vi "Station Class Server.vi"() -> ()   [LabVIEW 2018, in "Station.lvclass"]
uses:
  Station.lvclass
  Controls/Server Control.ctl
panel:
  in  "Stop Server":bool
  in  "Delete Ref":bool
  in  "Open References":i32(listbox)
  in  "Lock Server":bool
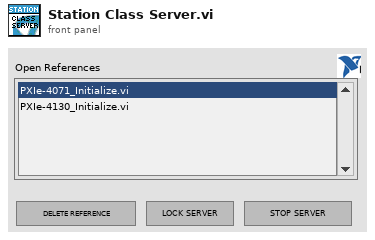
[diagram p1: front panel]
types:
  T1 = typedef "Server Control.ctl" = enum16{"Open New Reference", "Remove Reference", "Kill Server", "Set Station Ref", "Get Station Ref"}
  T2 = cluster{"Action (0: Create)":T1, "Creator Path (=\"\")":path, "Station in":refnum<class "Station.lvclass">}
  T3 = typedef "LVRectTypeDef.ctl" = cluster{"Left":i16, "Top":i16, "Right":i16, "Bottom":i16}
  T4 = cluster{"Action (0: Create)":T1, path, "Station in":refnum<class "Station.lvclass">}
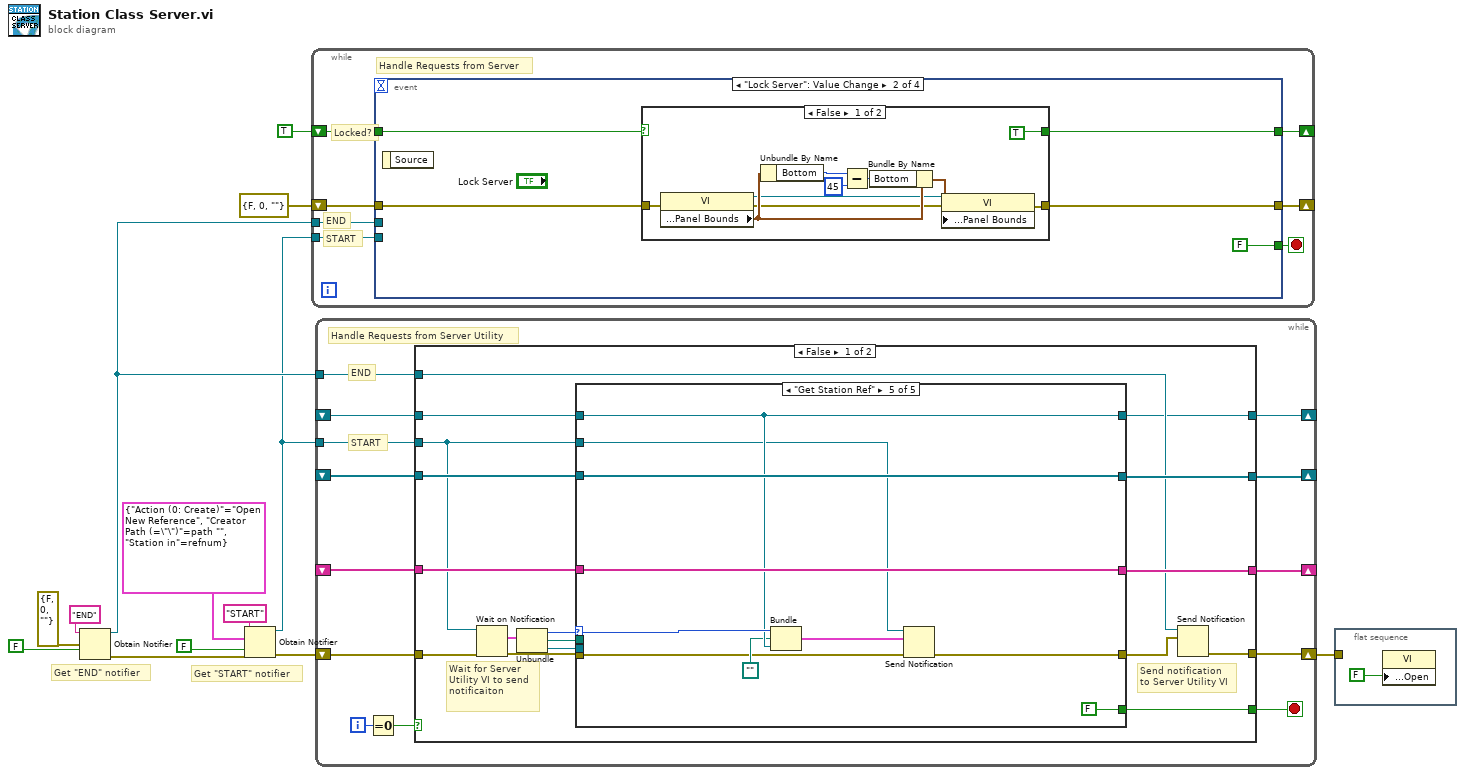
[diagram p0: block diagram]
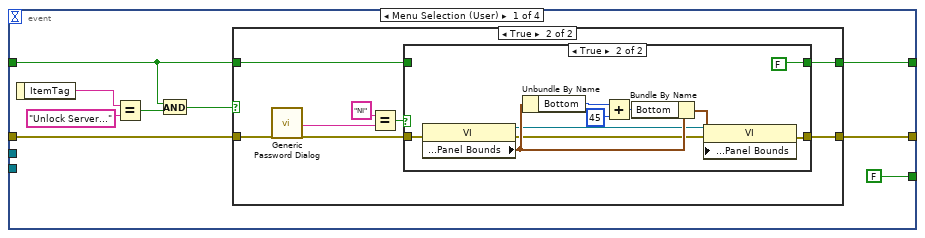
[diagram p2: hidden frame]
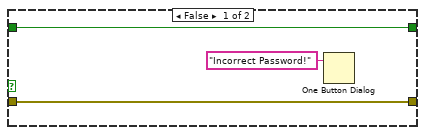
[diagram p4: hidden frame]
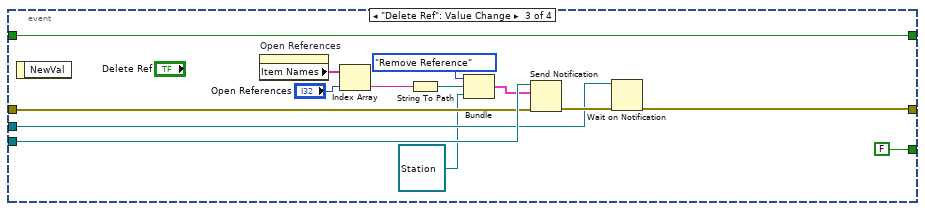
[diagram p6: hidden frame]
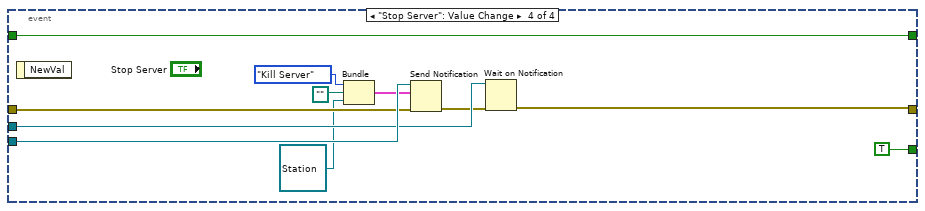
[diagram p7: hidden frame]
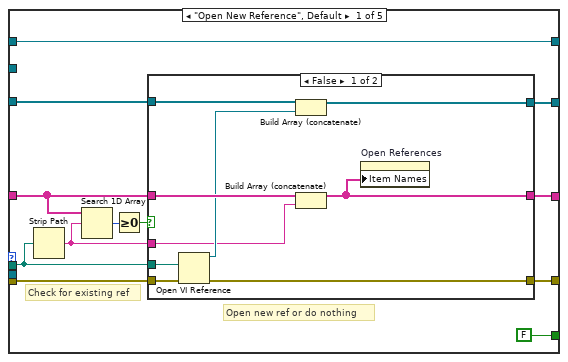
[diagram p8: hidden frame]
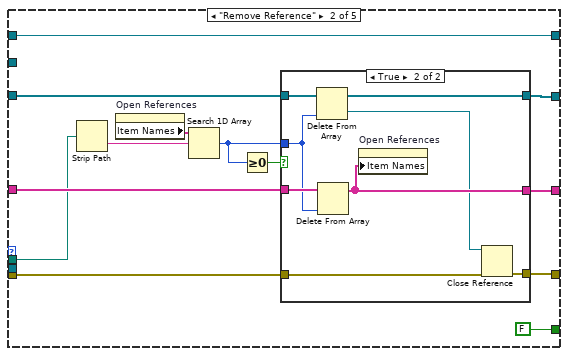
[diagram p10: hidden frame]
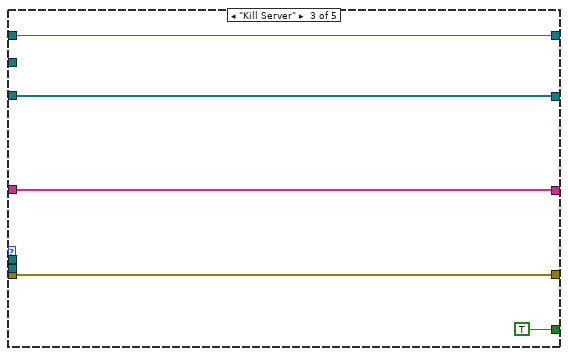
[diagram p12: hidden frame]
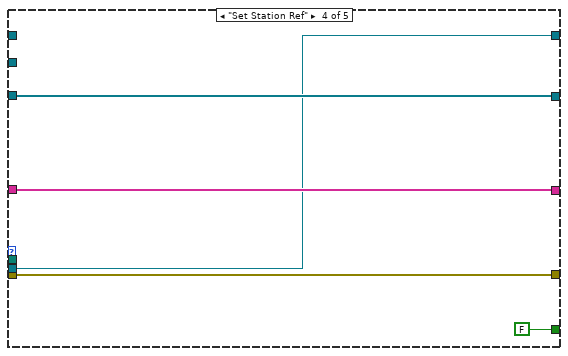
[diagram p13: hidden frame]
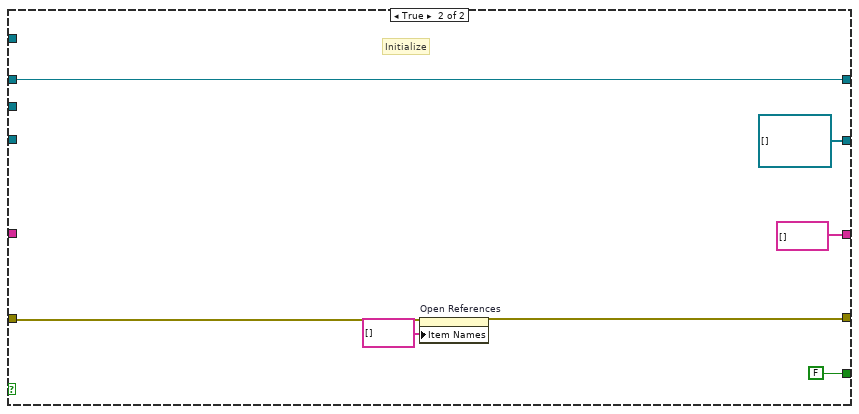
[diagram p14: hidden frame]
diagram:
  # "Get \"START\" notifier"
  # "Get \"END\" notifier"
  n1 = Obtain Notifier(name (unnamed)="END", notification data type=errorcluster {"status"=FALSE, "code"=0, "source"=""} ("error out"), create if not found? (T)=FALSE) -> (notifier out=w6:refnum<notifier>, error out=w7:errorcluster)  [unwired: 1 in, 1 out]
  n2 = Obtain Notifier(name (unnamed)="START", notification data type=T2 {"Action (0: Create)"=enum."Open New Reference", "Creator Path (=\"\")"=path "", "Station in"=refnum} ("output cluster"), create if not found? (T)=FALSE, error in (no error)=w7) -> (notifier out=w1:refnum<notifier>, error out=w5:errorcluster)  [unwired: 1 out]
  n3 = while {
    shift-right: [w18] -> _
    shift-left: errorcluster {"status"=FALSE, "code"=0, "source"=""} ("error out") -> [w19]
    tunnel: w6 -> [w17]
    tunnel: w1 -> [w16]
    shift-right: [w14] -> _
    shift-left: TRUE -> [w15]
    stop <- w20 stop-if-true
    # "Locked?"
    # "Handle Requests from Server"
    # "START"
    # "END"
    n4 = event shown="[1] \"Lock Server\": Value Change" {
      selector: _ -> [_ _ _ _]
      dyn-events: _ -> [_ _ _ _]
      timeout: _ -> [_ _ _ _]
      tunnel: [FALSE FALSE FALSE TRUE] -> w20
      tunnel: w19 -> [w26 w54 w82 w93]
      tunnel: [w25 w56 w72 w86] -> w18
      tunnel: w17 -> [_ _ w73 w88]
      tunnel: w16 -> [_ _ w83 w94]
      tunnel: w15 -> [w22 w53 w71 w85]
      tunnel: [w24 w55 w71 w85] -> w14
      event Menu Selection (User) {
        n5 = event-data() -> ("ItemTag"=w29:string)  [unwired: 1 in]
        n6 = Equal?(x=w29, y="Unlock Server...") -> (x = y?=w23:bool)
        n7 = And(x=w22, y=w23) -> (x .and. y?=w21:bool)
        n8 = case shown="True" w21 {
          tunnel: w26 -> [w31 w39]
          tunnel: [w31 w36] -> w25
          tunnel: [w30 w34] -> w24
          tunnel: w22 -> [w30 w33]
          frame False {
          }
          frame True {
            n9 = call "Generic Password Dialog.vi"("error in (no error)"=w39) -> ("Password:out"=w32:string, "error out"=w37:errorcluster)  [unwired: 16 in, 1 out]
            n10 = Equal?(x="NI", y=w32) -> (x = y?=w35:bool)
            n11 = case shown="True" w35 {
              tunnel: w37 -> [w41 w52]
              tunnel: [w41 w44] -> w36
              tunnel: w33 -> [w40 _]
              tunnel: [w40 FALSE] -> w34
              frame False {
                n12 = One Button Dialog(message="Incorrect Password!") -> ()  [unwired: 1 in, 1 out]
              }
              frame True {
                n13 = property class="VI"(error in=w52) -> (reference out=w47:refnum<vi>, error out=w46:errorcluster, "Front Panel Window:Panel Bounds"=w51:T3)  [unwired: 1 in]
                n14 = Unbundle By Name(w51) -> ("Bottom"=w50:i16)
                n15 = Add(x=w50, y=i16 45) -> (x+y=w48:i16)
                n16 = Bundle By Name(cluster=w51, "Bottom"=w48) -> (w45:T3)
                n17 = property class="VI"(reference=w47, error in=w46, "Front Panel Window:Panel Bounds"=w45) -> (error out=w44:errorcluster)  [unwired: 1 out]
              }
            }
          }
        }
      }
      event "Lock Server": Value Change {
        n18 = event-data() -> ()  [unwired: 1 in, 1 out]
        n19 = case shown="False" w53 {
          selector: w53 -> [_ w69]
          tunnel: w54 -> [w67 w68]
          tunnel: [w59 w68] -> w56
          tunnel: [TRUE w69] -> w55
          frame False {
            n20 = property class="VI"(error in=w67) -> (reference out=w62:refnum<vi>, error out=w61:errorcluster, "Front Panel Window:Panel Bounds"=w66:T3)  [unwired: 1 in]
            n21 = Unbundle By Name(w66) -> ("Bottom"=w65:i16)
            n22 = Subtract(x=w65, y=i16 45) -> (x-y=w63:i16)
            n23 = Bundle By Name(cluster=w66, "Bottom"=w63) -> (w60:T3)
            n24 = property class="VI"(reference=w62, error in=w61, "Front Panel Window:Panel Bounds"=w60) -> (error out=w59:errorcluster)  [unwired: 1 out]
          }
          frame True {
          }
        }
      }
      event "Delete Ref": Value Change {
        n25 = event-data() -> ()  [unwired: 1 in, 1 out]
        n26 = property on="Open References" class="LstBox (strict)"() -> ("Item Names"=w80:string[])  [unwired: 2 in, 2 out]
        n27 = Index Array(array=w80, index="Open References") -> (element=w78:string)
        n28 = String To Path(string=w78) -> (path=w76:path)
        n29 = Bundle("Action (0: Create)"=Server_Control."Remove Reference", w76, "Station in"=refnum<class "Station.lvclass"> refnum) -> (w77:T4)  [unwired: 1 in]
        n30 = Send Notification(notification=w77, notifier=w83, error in (no error)=w82) -> (error out=w74:errorcluster)  [unwired: 1 out]
        n31 = Wait on Notification(notifier=w73, error in (no error)=w74) -> (error out=w72:errorcluster)  [unwired: 2 in, 3 out]
      }
      event "Stop Server": Value Change {
        n32 = event-data() -> ()  [unwired: 1 in, 1 out]
        n33 = Bundle("Action (0: Create)"=Server_Control."Kill Server", path "", "Station in"=refnum<class "Station.lvclass"> refnum) -> (w91:T4)  [unwired: 1 in]
        n34 = Send Notification(notification=w91, notifier=w94, error in (no error)=w93) -> (error out=w87:errorcluster)  [unwired: 1 out]
        n35 = Wait on Notification(notifier=w88, error in (no error)=w87) -> (error out=w86:errorcluster)  [unwired: 2 in, 3 out]
      }
    }
  }
  n36 = while {
    shift-right: [w106] -> _
    shift-left: _ -> [w107]
    shift-right: [w100] -> w3
    shift-left: w5 -> [w103]
    shift-right: [w105] -> _
    shift-left: _ -> [w104]
    tunnel: w6 -> [w99]
    tunnel: w1 -> [w102]
    shift-right: [w96] -> _
    shift-left: _ -> [w95]
    i -> [w97]
    stop <- w101 stop-if-true
    # "Handle Requests from Server Utility"
    # "START"
    # "END"
    n37 = Equal To 0?(x=w97) -> (x = 0?=w98:bool)
    n38 = case shown="False" w98 {
      tunnel: w107 -> [w124 _]
      tunnel: [w123 refnum<vi>[] []] -> w106
      tunnel: [w122 string[] []] -> w105
      tunnel: w104 -> [w121 _]
      tunnel: w103 -> [w116 w198]
      tunnel: w102 -> [w108 _]
      tunnel: [w115 FALSE] -> w101
      tunnel: [w113 w194] -> w100
      tunnel: w99 -> [w112 _]
      tunnel: [w110 w193] -> w96
      tunnel: w95 -> [w109 w193]
      frame False {
        # "Send notification to Server Utility VI"
        # "Wait for Server Utility VI to send notificaiton"
        n39 = Wait on Notification(notifier=w108, error in (no error)=w116) -> (notification=w120:T2, error out=w119:errorcluster)  [unwired: 2 in, 2 out]
        n40 = Unbundle(w120) -> ("Action (0: Create)"=w118:T1, "Creator Path (=\"\")"=w117:path, "Station in"=w111:refnum<class "Station.lvclass">)
        n41 = case shown="\"Get Station Ref\"" w118 {
          selector: w118 -> [_ _ _ _ w188]
          tunnel: w124 -> [w135 w158 w177 w182 w192]
          tunnel: w119 -> [w136 w156 w176 w181 w185]
          tunnel: [w131 w155 w176 w181 w189] -> w114
          tunnel: [w134 w160 w177 w182 w192] -> w123
          tunnel: w117 -> [w129 w154 _ _ _]
          tunnel: [w127 w157 w175 w180 w191] -> w122
          tunnel: w121 -> [w128 w159 w175 w180 w191]
          tunnel: [FALSE FALSE TRUE FALSE FALSE] -> w115
          tunnel: w111 -> [_ _ _ w178 _]
          tunnel: [w125 w149 w173 w178 w187] -> w110
          tunnel: w109 -> [w125 w149 w173 _ w187]
          tunnel: w108 -> [_ _ _ _ w184]
          frame "Open New Reference", Default {
            # "Open new ref or do nothing"
            # "Check for existing ref"
            n42 = Strip Path(path=w129) -> (name=w126:string)  [unwired: 1 out]
            n43 = Search 1D Array(1D array=w128, element=w126) -> (index of element=w132:i32)  [unwired: 1 in]
            n44 = Greater Or Equal To 0?(x=w132) -> (x >= 0?=w133:bool)
            n45 = case shown="False" w133 {
              tunnel: w136 -> [w145 w148]
              tunnel: [w144 w148] -> w131
              tunnel: w135 -> [w143 w147]
              tunnel: [w142 w147] -> w134
              tunnel: w129 -> [w141 _]
              tunnel: w128 -> [w140 w146]
              tunnel: [w138 w146] -> w127
              tunnel: w126 -> [w137 _]
              frame False {
                n46 = Open VI Reference(vi path=w141, error in (no error)=w145) -> (vi reference=w139:refnum<vi>, error out=w144:errorcluster)  [unwired: 4 in]
                n47 = Build Array (concatenate)(w143, w139) -> (w142:refnum<vi>[])
                n48 = Build Array (concatenate)(w140, w137) -> (w138:string[])
                n49 = property on="Open References" class="LstBox (strict)"("Item Names"=w138) -> ()  [unwired: 2 in, 2 out]
              }
              frame True {
              }
            }
          }
          frame "Remove Reference" {
            n50 = Strip Path(path=w154) -> (name=w152:string)  [unwired: 1 out]
            n51 = property on="Open References" class="LstBox (strict)"() -> ("Item Names"=w153:string[])  [unwired: 2 in, 2 out]
            n52 = Search 1D Array(1D array=w153, element=w152) -> (index of element=w150:i32)  [unwired: 1 in]
            n53 = Greater Or Equal To 0?(x=w150) -> (x >= 0?=w151:bool)
            n54 = case shown="True" w151 {
              tunnel: w158 -> [w164 w172]
              tunnel: [w164 w171] -> w160
              tunnel: w159 -> [w163 w170]
              tunnel: [w163 w168] -> w157
              tunnel: w150 -> [_ w169]
              tunnel: w156 -> [w162 w167]
              tunnel: [w162 w166] -> w155
              frame False {
              }
              frame True {
                n55 = Delete From Array(array=w172, index=w169) -> (deleted portion=w165:refnum<vi>, array with subset deleted=w171:refnum<vi>[])  [unwired: 1 in]
                n56 = Delete From Array(array=w170, index=w169) -> (array with subset deleted=w168:string[])  [unwired: 1 in, 1 out]
                n57 = property on="Open References" class="LstBox (strict)"("Item Names"=w168) -> ()  [unwired: 2 in, 2 out]
                n58 = Close Reference(reference=w165, error in (no error)=w167) -> (error out=w166:errorcluster)
              }
            }
          }
          frame "Kill Server" {
          }
          frame "Set Station Ref" {
          }
          frame "Get Station Ref" {
            n59 = Bundle("Action (0: Create)"=w188, path "", "Station in"=w187) -> (w183:T4)  [unwired: 1 in]
            n60 = Send Notification(notification=w183, notifier=w184, error in (no error)=w185) -> (error out=w189:errorcluster)  [unwired: 1 out]
          }
        }
        n61 = Send Notification(notification=w114, notifier=w112) -> (error out=w113:errorcluster)  [unwired: 1 in, 1 out]
      }
      frame True {
        # "Initialize"
        n62 = property on="Open References" class="LstBox (strict)"(error in=w198, "Item Names"=string[] []) -> (error out=w194:errorcluster)  [unwired: 1 in, 1 out]
      }
    }
  }
  n63 = flat-sequence {
    tunnel: w3 -> [_]
    frame #0 {
      n64 = property class="VI"("Front Panel Window:Open"=FALSE) -> ()  [unwired: 2 in, 2 out]
    }
  }
